vi "ASK-DEMOD.vi"() -> ()   [LabVIEW 2012]
panel:
  out "Demodulated Graph":dynamicdata(graph)
  in  "baseband":dbl(slide) scale=0.0..500.0
  in  "carr":dbl(slide) scale=0.0..2000.0
  in  "lower-cutoff":dbl
  out "ASK":dynamicdata(graph)
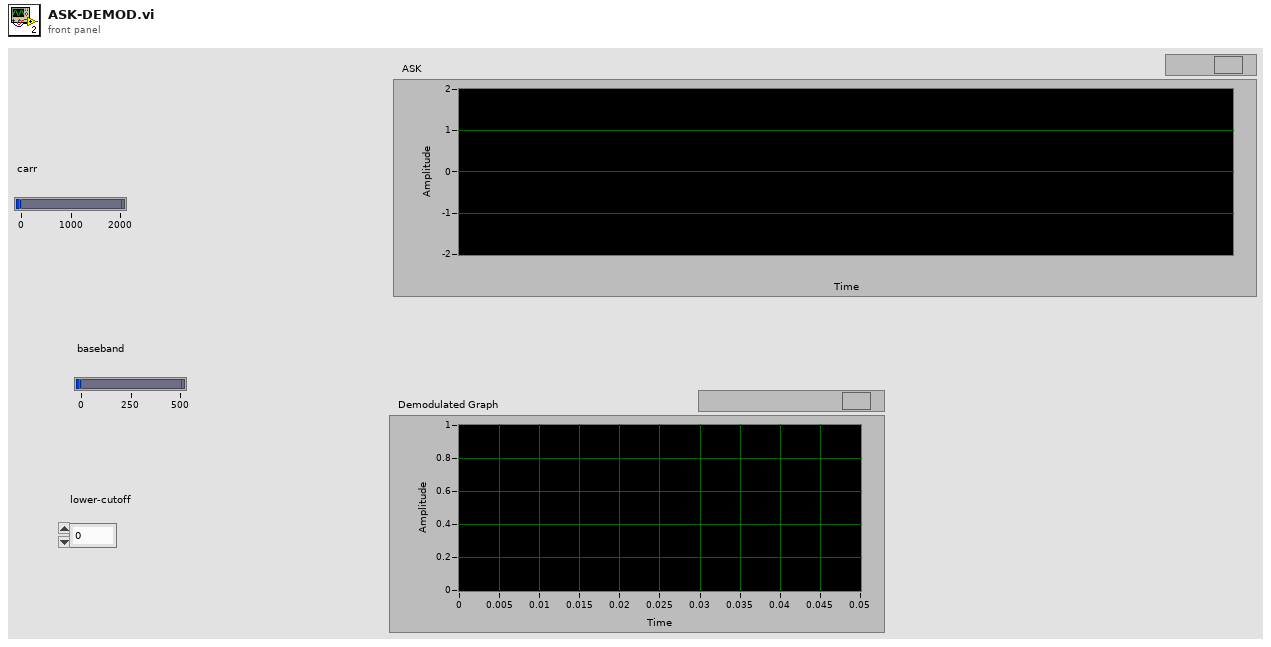
[diagram p1: front panel]
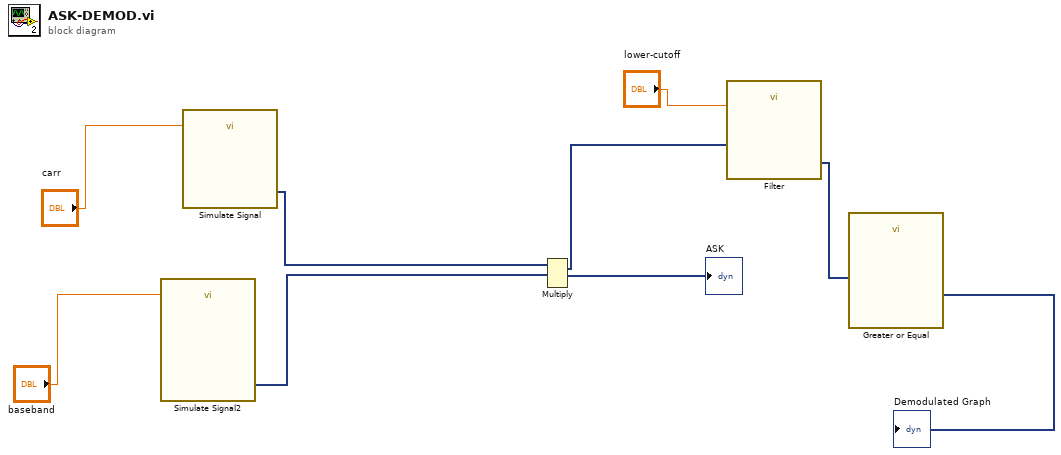
[diagram p0: block diagram]
diagram:
  n1 = call "Simulate Signal2"("Frequency"="baseband") -> ("Square"=w7:dynamicdata)  [unwired: 13 in, 1 out]
  n2 = call "Simulate Signal"("Frequency"="carr") -> ("Sine"=w8:dynamicdata)  [unwired: 13 in, 1 out]
  n3 = Multiply(1:w7, 2:w8) -> (0:w6:dynamicdata)  [unwired: 1 in, 1 out]
  "ASK" <- w6
  n4 = call "Filter"("Lower Cut-Off"="lower-cutoff", "Signal"=w6) -> ("Filtered Signal"=w5:dynamicdata)  [unwired: 8 in, 1 out]
  n5 = call "Greater or Equal"("Operand 1"=w5) -> ("Result"=→"Demodulated Graph":dynamicdata)  [unwired: 9 in, 1 out]
